vi "CélulaDessalinizadora3.0.vi"() -> ()   [LabVIEW 2014]
panel:
  in  "Adsorção":bool
  in  "OK Button":bool
  in  "Documento de Texto":path
  out "Tempo":dbl
  in  "Condutividade Máxima":dbl
  in  "NÚMERO DE CICLOS":dbl
  in  "Liga/Desliga":bool
  in  "Escolha: Porta Serial":refnum<visa-resource-name>="COM3"
  out "Dessorção":bool
  out "Adsorção":bool
  out "Single-Pass":bool
  out "Batch":bool
  in  "BATCH / SINGLE PASS":bool
  out "Potencial de Célula [mV]":dbl(graph)
  out "pH":dbl(graph)
  out "Condutividade [us/cm]":dbl(graph)
  in  "Selecionar caso":T1(tab)
  in  "TEMPO DE ADSOR敲O P":dbl
  in  "CONDUTIVIDADE \nMÍNIMA NA ADSORÇÃO P":dbl
  in  "TEMPO DE DESSOR敲O P":dbl
  in  "CONDUTIVIDADE \nMÁXIMA NA DESSORÇÃO P":dbl
  in  "Selecionar parâmetro G":enum32{"Tempo", "Condutividade", "Potencial"}(tab)
  in  "TEMPO DE ADSOR敲O G":dbl
  in  "TEMPO DE DESSOR敲O G":dbl
  in  "CONDUTIVIDADE \nMÍNIMA NA ADSORÇÃO G":dbl
  in  "CONDUTIVIDADE \nMÁXIMA NA DESSORÇÃO G":dbl
  in  "POTENCIAL DE CORTE\nNA ADSOR敲O":dbl
  in  "POTENCIAL DE CORTE\nNA DESSOR敲O":dbl
  in  "POTENCIAL DE CORTE\nNA DESSOR敲O G":dbl
  in  "CONDUTIVIDADE \nMÁXIMA NA DESSORÇÃO G2":dbl
  in  "TEMPO DE DESSOR敲O G 2":dbl
  in  "TEMPO DE ADSOR敲O G 2":dbl
  in  "CONDUTIVIDADE \nMÍNIMA NA ADSORÇÃO G 2":dbl
  in  "POTENCIAL DE CORTE\nNA ADSOR敲O G":dbl
  # "CONDUTIVIDADE MÁXIMA"
  # "s"
  # "us/cm"
  # "s"
  # "us/cm"
  # "s"
  # "s"
  # "us/cm"
  # "us/cm"
  # "VV"
  # "V"
  # "s"
  # "us/cm"
  # "mV"
  # "s"
  # "us/cm"
  # "mV"
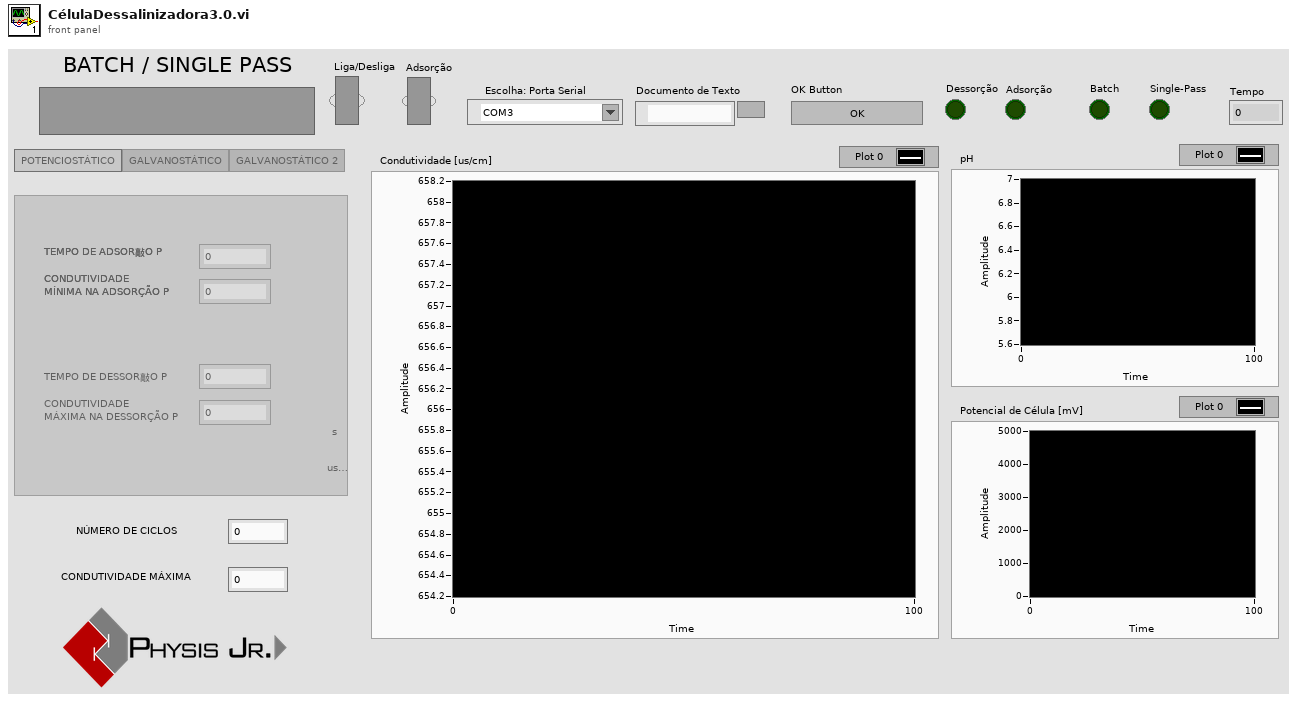
[diagram p1: front panel]
types:
  T1 = enum32{"POTENCIOSTÁTICO", "GALVANOSTÁTICO", "GALVANOSTÁTICO 2"}
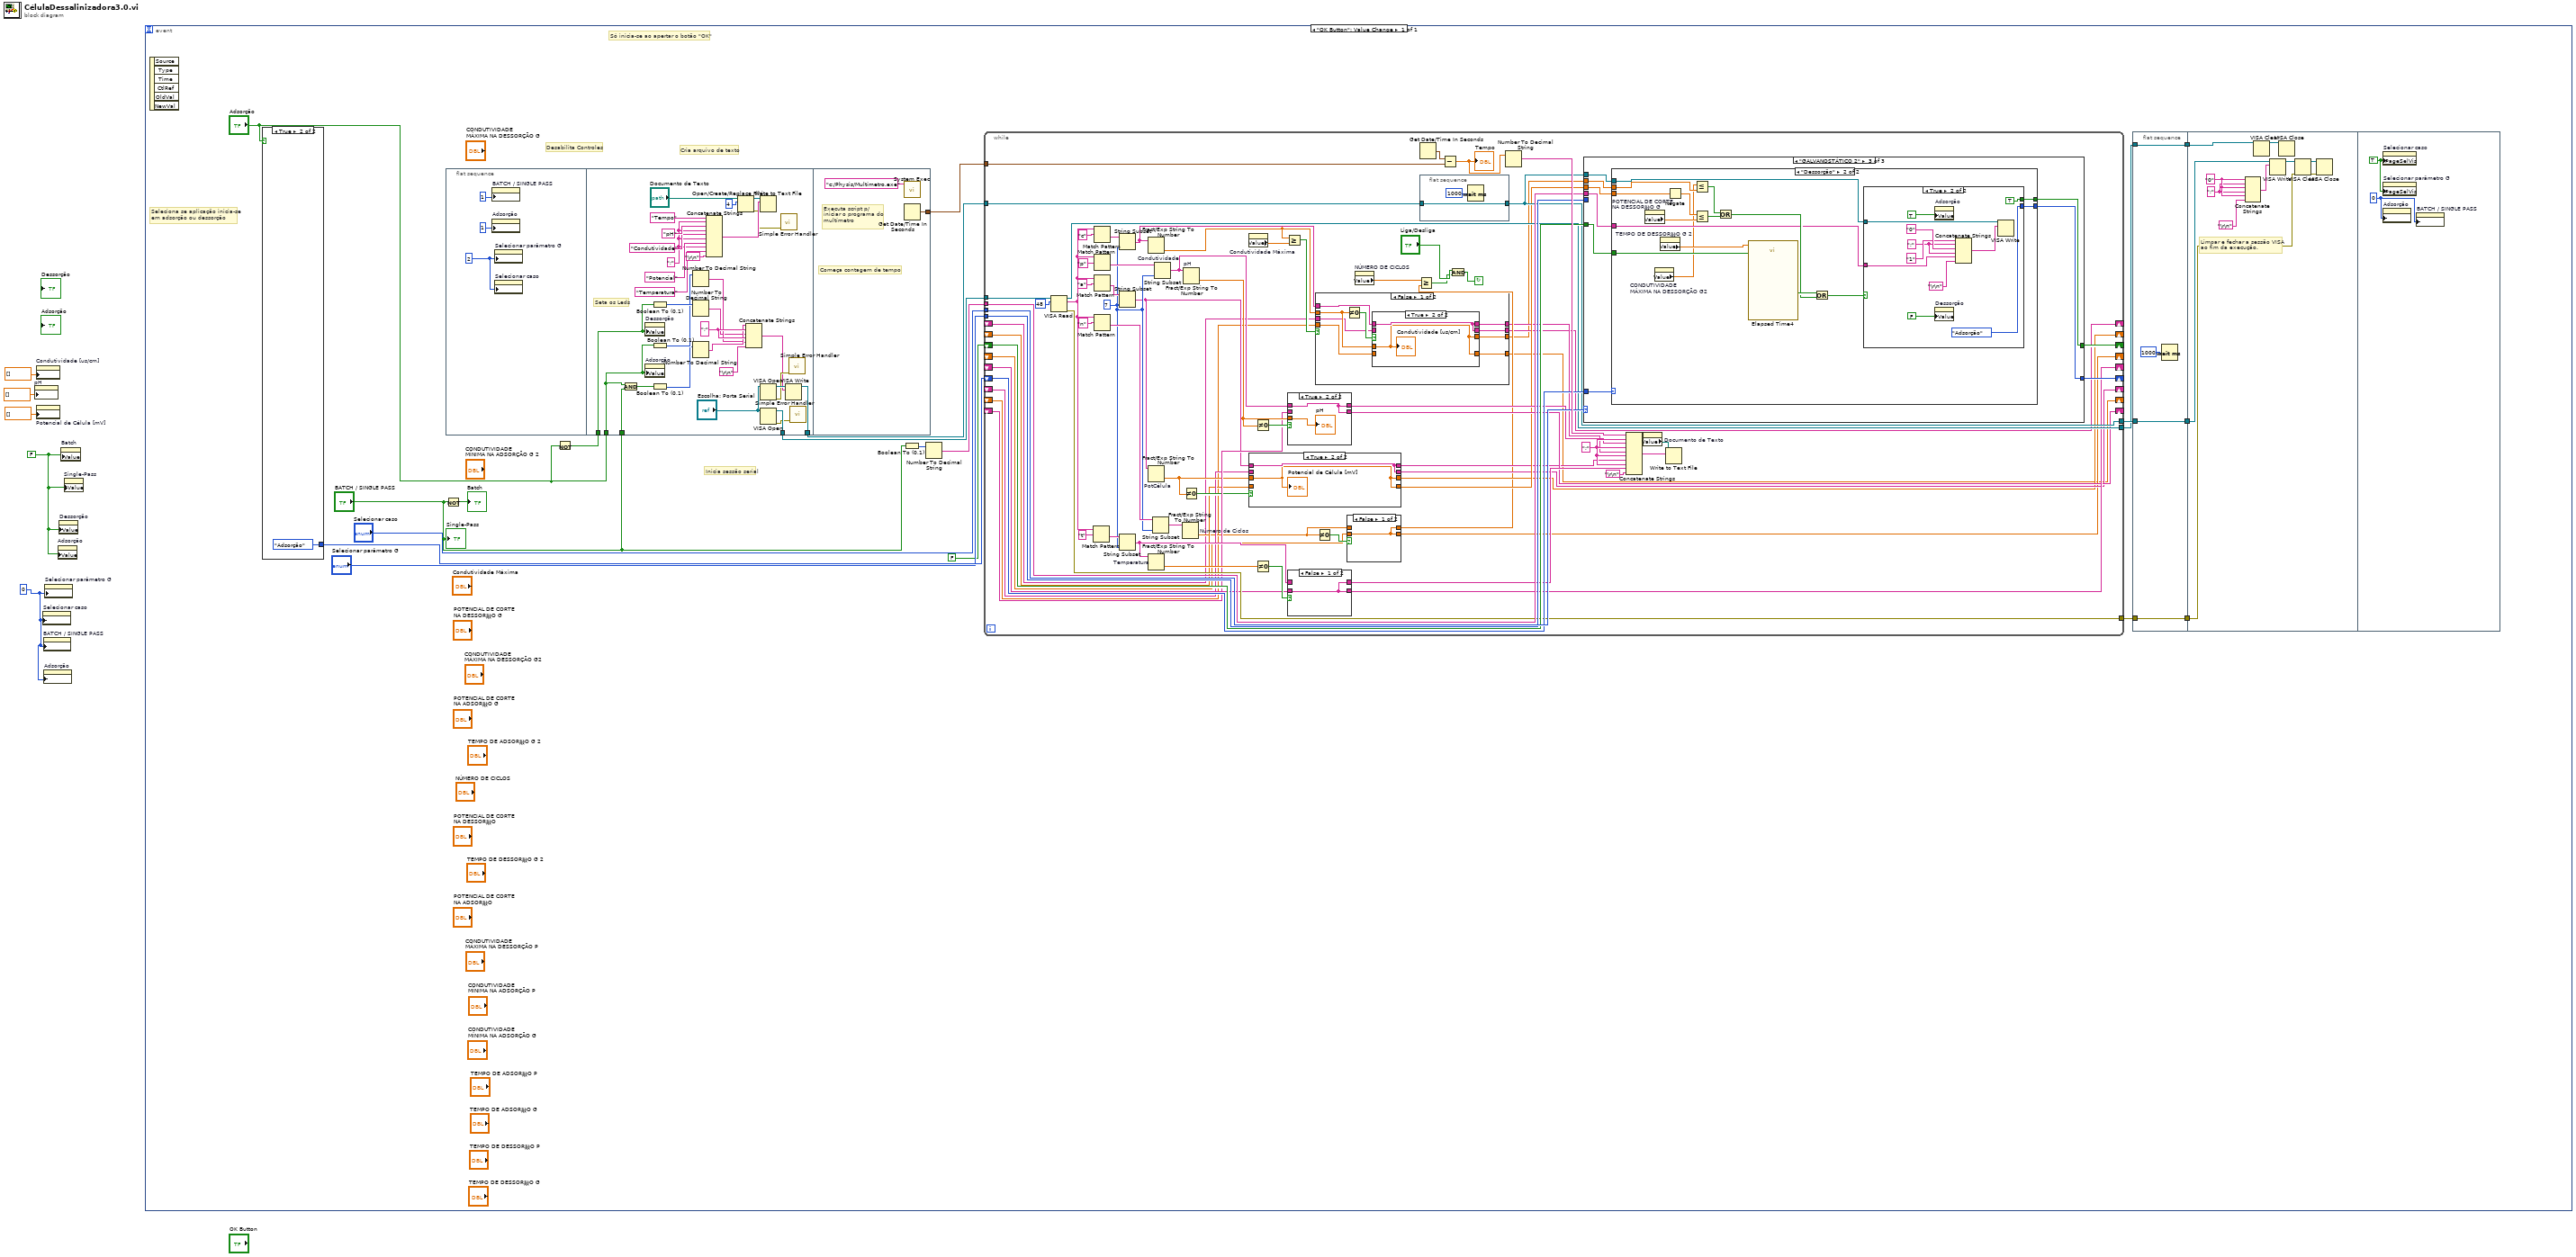
[diagram p0: block diagram]
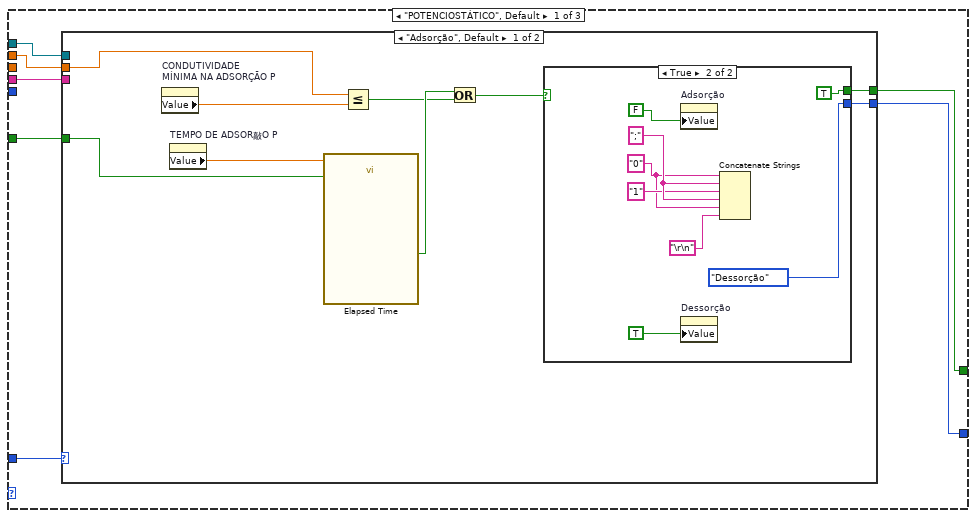
[diagram p6: hidden frame]
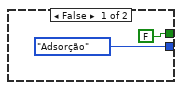
[diagram p7: hidden frame]
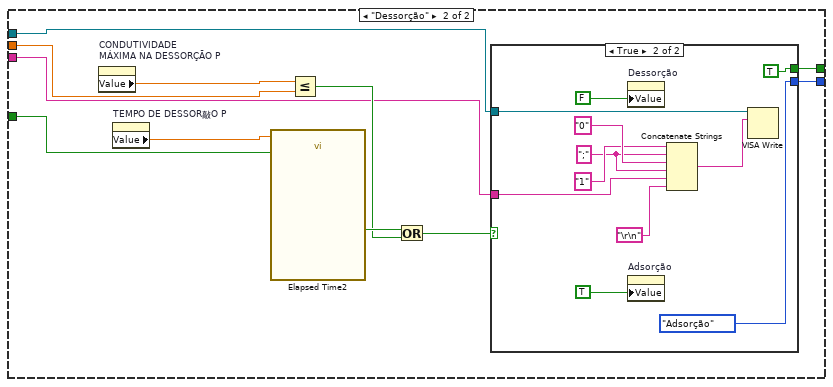
[diagram p8: hidden frame]
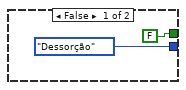
[diagram p9: hidden frame]
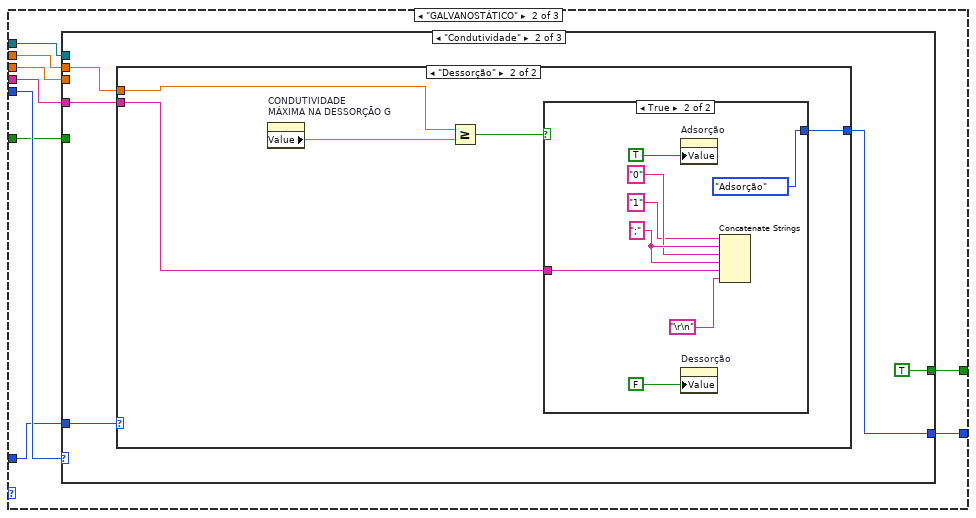
[diagram p10: hidden frame]
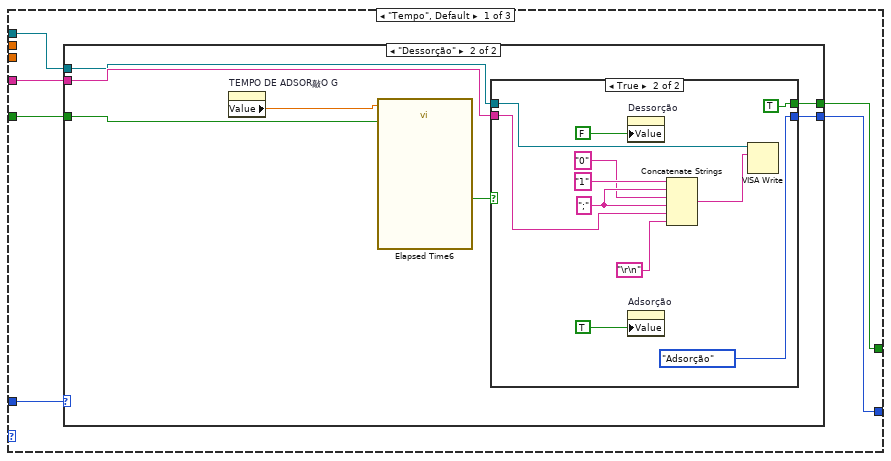
[diagram p11: hidden frame]
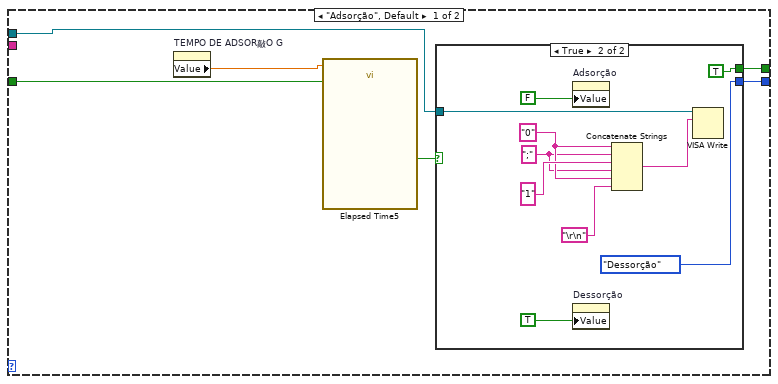
[diagram p12: hidden frame]
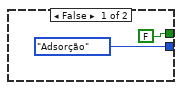
[diagram p13: hidden frame]
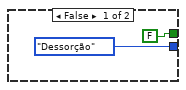
[diagram p14: hidden frame]
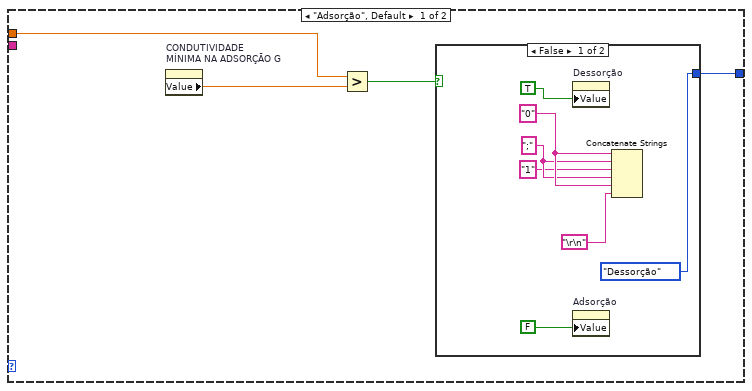
[diagram p15: hidden frame]
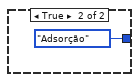
[diagram p16: hidden frame]
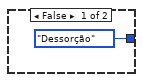
[diagram p17: hidden frame]
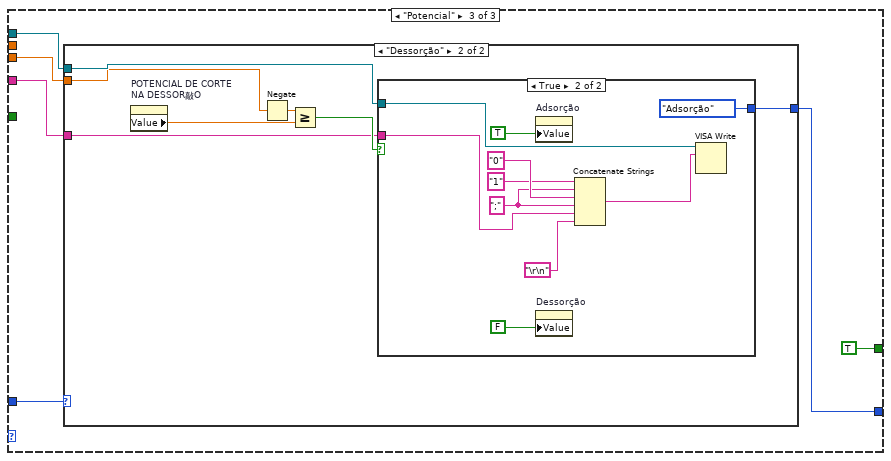
[diagram p18: hidden frame]
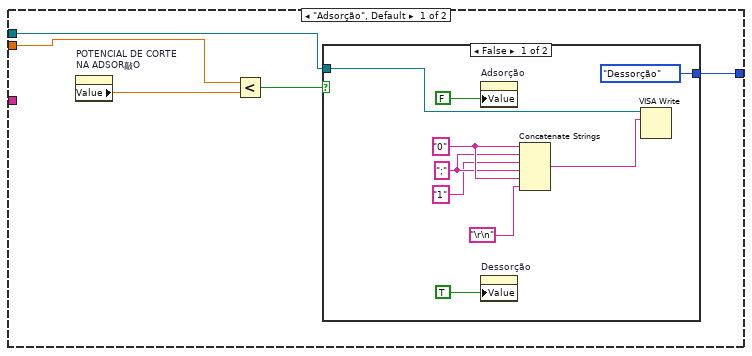
[diagram p19: hidden frame]
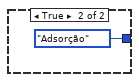
[diagram p20: hidden frame]
diagram:
  w1 = 0
  w2 = FALSE
  n1 = property on="pH" class="WFChart (strict)"("History Data"=dbl[] []) -> ()  [unwired: 2 in, 2 out]
  n2 = property on="Condutividade [us/cm]" class="WFChart (strict)"("History Data"=dbl[] []) -> ()  [unwired: 2 in, 2 out]
  n3 = property on="Potencial de Célula [mV]" class="WFChart (strict)"("History Data"=dbl[] []) -> ()  [unwired: 2 in, 2 out]
  n4 = property on="Selecionar caso" class="TabCtl (strict)"("DisabledEnum"=w1) -> ()  [unwired: 2 in, 2 out]
  n5 = property on="BATCH / SINGLE PASS" class="Bool (strict)"("DisabledEnum"=w1) -> ()  [unwired: 2 in, 2 out]
  n6 = property on="Adsorção" class="Bool (strict)"("DisabledEnum"=w1) -> ()  [unwired: 2 in, 2 out]
  n7 = property on="Selecionar parâmetro G" class="TabCtl (strict)"("DisabledEnum"=w1) -> ()  [unwired: 2 in, 2 out]
  n8 = property on="Adsorção" class="Bool (strict)"("Value"=w2) -> ()  [unwired: 2 in, 2 out]
  n9 = property on="Dessorção" class="Bool (strict)"("Value"=w2) -> ()  [unwired: 2 in, 2 out]
  n10 = property on="Batch" class="Bool (strict)"("Value"=w2) -> ()  [unwired: 2 in, 2 out]
  n11 = property on="Single-Pass" class="Bool (strict)"("Value"=w2) -> ()  [unwired: 2 in, 2 out]
  n12 = event shown="[0] \"OK Button\": Value Change" {
    selector: _ -> [_]
    dyn-events: _ -> [_]
    timeout: _ -> [_]
    event "OK Button": Value Change {
      # "Inicia sessão serial"
      # "Cria arquivo de texto"
      # "Desabilita Controles"
      # "Só inicia-se ao apertar o botão \"OK\""
      # "Seleciona se aplicação inicia-se\nem adsorção ou dessorção"
      n13 = event-data() -> ()  [unwired: 1 in, 6 out]
      n14 = case shown="True" "Adsorção" {
        tunnel: [enum16{"Adsorção", "Dessorção"}."Dessorção" enum16{"Adsorção", "Dessorção"}."Adsorção"] -> w18
        frame False {
        }
        frame True {
        }
      }
      n15 = Not(x="BATCH / SINGLE PASS") -> (.not. x?=→"Batch":bool)
      n16 = flat-sequence {
        tunnel: "Adsorção" -> [w47]
        tunnel: w16 -> [w56]
        tunnel: "BATCH / SINGLE PASS" -> [w59]
        tunnel: [w55] -> w11
        tunnel: [w54] -> w10
        tunnel: [w77] -> w15
        frame #0 {
          w42 = 2
          n17 = property on="BATCH / SINGLE PASS" class="Bool (strict)"("DisabledEnum"=1) -> ()  [unwired: 2 in, 2 out]
          n18 = property on="Adsorção" class="Bool (strict)"("DisabledEnum"=1) -> ()  [unwired: 2 in, 2 out]
          n19 = property on="Selecionar parâmetro G" class="TabCtl (strict)"("DisabledEnum"=w42) -> ()  [unwired: 2 in, 2 out]
          n20 = property on="Selecionar caso" class="TabCtl (strict)"("DisabledEnum"=w42) -> ()  [unwired: 2 in, 2 out]
        }
        frame #1 {
          w63 = ";"
          w67 = ";"
          # "Seta os Leds"
          n21 = And(x=w47, y=w59) -> (x .and. y?=w58:bool)
          n22 = property on="Dessorção" class="Bool (strict)"("Value"=w56) -> ()  [unwired: 2 in, 2 out]
          n23 = property on="Adsorção" class="Bool (strict)"("Value"=w47) -> ()  [unwired: 2 in, 2 out]
          n24 = Boolean To (0,1)(Boolean=w56) -> (0, 1=w61:i16)
          n25 = Boolean To (0,1)(Boolean=w47) -> (0, 1=w60:i16)
          n26 = Boolean To (0,1)(Boolean=w58) -> (0, 1=w57:i16)
          n27 = Number To Decimal String(number=w60) -> (decimal integer string=w49:string)  [unwired: 1 in]
          n28 = Number To Decimal String(number=w61) -> (decimal integer string=w48:string)  [unwired: 1 in]
          n29 = Number To Decimal String(number=w57) -> (decimal integer string=w50:string)  [unwired: 1 in]
          n30 = Concatenate Strings("Tempo", w67, "pH", w67, "Condutividade", w67, "Potencial", w67, "Temperatura", "\r\n") -> (w65:string)
          n31 = Open/Create/Replace File(file path (use dialog)="Documento de Texto", operation (0:open)=4) -> (refnum out=w73:refnum<file>, error out=w53:errorcluster)  [unwired: 4 in, 1 out]
          n32 = Concatenate Strings(w50, w63, w48, w63, w49, "\r\n") -> (w46:string)
          n33 = Write to Text File(file (use dialog)=w73, text=w65) -> ()  [unwired: 2 in, 3 out]
          n34 = VISA Open(VISA resource name="Escolha: Porta Serial") -> (VISA resource name=w62:refnum<visa-resource-name>, error out=w52:errorcluster)  [unwired: 4 in]
          n35 = VISA Open(VISA resource name="Escolha: Porta Serial") -> (VISA resource name=w55:refnum<visa-resource-name>, error out=w51:errorcluster)  [unwired: 4 in]
          n36 = call <vilib>:"Simple Error Handler.vi"("error in (no error)"=w53) -> ()  [unwired: 4 in, 5 out]
          n37 = VISA Write(VISA resource name=w62, write buffer=w46) -> (VISA resource name out=w54:refnum<visa-resource-name>)  [unwired: 1 in, 2 out]
          n38 = call <vilib>:"Simple Error Handler.vi"("error in (no error)"=w52) -> ()  [unwired: 4 in, 5 out]
          n39 = call <vilib>:"Simple Error Handler.vi"("error in (no error)"=w51) -> ()  [unwired: 4 in, 5 out]
        }
        frame #2 {
          # "Executa script p/\niniciar o programa do\nmultímetro"
          # "Começa contagem de tempo"
          n40 = call <vilib>:"System Exec.vi"("command line"="c:/Physis/Multímetro.exe") -> ()  [unwired: 7 in, 4 out]
          n41 = Get Date/Time In Seconds() -> (seconds since 1Jan1904=w77:timestamp)
        }
      }
      n42 = Not(x="Adsorção") -> (.not. x?=w16:bool)
      n43 = Boolean To (0,1)(Boolean="BATCH / SINGLE PASS") -> (0, 1=w13:i16)
      n44 = Number To Decimal String(number=w13) -> (decimal integer string=w12:string)  [unwired: 1 in]
      n45 = while {
        tunnel: w11 -> [w150]
        tunnel: w15 -> [w128]
        tunnel: "Selecionar caso" -> [w127]
        shift-right: [w126] -> _
        shift-left: w18 -> [w125]
        shift-right: [w124] -> _
        shift-left: FALSE -> [w123]
        tunnel: w12 -> [w122]
        tunnel: w10 -> [w120]
        tunnel: "Selecionar parâmetro G" -> [w121]
        tunnel: [w119] -> w9
        tunnel: [w118] -> w8
        tunnel: [w117] -> w7
        shift-right: [w110] -> _
        shift-left: _ -> [w109]
        shift-right: [w104] -> _
        shift-left: _ -> [w103]
        shift-right: [w97] -> _
        shift-left: _ -> [w96]
        shift-right: [w95] -> _
        shift-left: _ -> [w94]
        shift-right: [w90] -> _
        shift-left: _ -> [w89]
        shift-right: [w86] -> _
        shift-left: _ -> [w85]
        shift-right: [w83] -> _
        shift-left: _ -> [w82]
        stop <- w78 continue-if-true
        w132 = ";"
        w139 = 7
        n46 = VISA Read(VISA resource name=w150, byte count=48) -> (VISA resource name out=w118:refnum<visa-resource-name>, read buffer=w137:string, error out=w117:errorcluster)  [unwired: 1 in, 1 out]
        n47 = Match Pattern(string=w137, regular expression="t") -> (after substring=w145:string)  [unwired: 1 in, 3 out]
        n48 = Match Pattern(string=w137, regular expression="c") -> (after substring=w140:string)  [unwired: 1 in, 3 out]
        n49 = Match Pattern(string=w137, regular expression="a") -> (after substring=w143:string)  [unwired: 1 in, 3 out]
        n50 = Match Pattern(string=w137, regular expression="p") -> (after substring=w144:string)  [unwired: 1 in, 3 out]
        n51 = Match Pattern(string=w137, regular expression="n") -> (after substring=w142:string)  [unwired: 1 in, 3 out]
        n52 = String Subset(string=w140, length (rest)=w139) -> (substring=w129:string)  [unwired: 1 in]
        n53 = String Subset(string=w143, length (rest)=w139) -> (substring=w99:string)  [unwired: 1 in]
        n54 = String Subset(string=w145, length (rest)=w139) -> (substring=w112:string)  [unwired: 1 in]
        n55 = Fract/Exp String To Number "Condutividade"(string=w129) -> (number=w88:dbl)  [unwired: 3 in, 1 out]
        n56 = Fract/Exp String To Number "PotCélula"(string=w99) -> (number=w101:dbl)  [unwired: 3 in, 1 out]
        n57 = Fract/Exp String To Number "Temperatura"(string=w112) -> (number=w114:dbl)  [unwired: 3 in, 1 out]
        n58 = String Subset(string=w142, length (rest)=w139) -> (substring=w138:string)  [unwired: 1 in]
        n59 = String Subset(string=w144, length (rest)=w139) -> (substring=w106:string)  [unwired: 1 in]
        n60 = Fract/Exp String To Number "Número de Ciclos"(string=w138) -> (number=w92:dbl)  [unwired: 3 in, 1 out]
        n61 = Fract/Exp String To Number "pH"(string=w106) -> (number=w107:dbl)  [unwired: 3 in, 1 out]
        n62 = Not Equal To 0?(x=w101) -> (x != 0?=w102:bool)
        n63 = property on="Condutividade Máxima" class="DigNum (strict)"() -> ("Value"=w116:dbl)  [unwired: 2 in, 2 out]
        n64 = case shown="True" w102 {
          tunnel: w101 -> [_ w156]
          tunnel: [w154 w156] -> w100
          tunnel: w99 -> [_ w157]
          tunnel: [w155 w157] -> w98
          tunnel: [w155 w157] -> w97
          tunnel: w96 -> [w155 _]
          tunnel: [w154 w156] -> w95
          tunnel: w94 -> [w154 _]
          frame False {
          }
          frame True {
            "Potencial de Célula [mV]" <- w156
          }
        }
        n65 = Not Equal To 0?(x=w107) -> (x != 0?=w108:bool)
        n66 = Not Equal To 0?(x=w114) -> (x != 0?=w113:bool)
        n67 = Greater Or Equal?(x=w88, y=w116) -> (x >= y?=w130:bool)
        n68 = case shown="True" w108 {
          tunnel: w107 -> [_ w160]
          tunnel: w106 -> [_ w159]
          tunnel: [w158 w159] -> w105
          tunnel: [w158 w159] -> w104
          tunnel: w103 -> [w158 _]
          frame False {
          }
          frame True {
            "pH" <- w160
          }
        }
        n69 = case shown="False" w113 {
          tunnel: w112 -> [_ w162]
          tunnel: [w161 w162] -> w111
          tunnel: [w161 w162] -> w110
          tunnel: w109 -> [w161 _]
          frame False {
          }
          frame True {
          }
        }
        n70 = case shown="False" w130 {
          tunnel: w129 -> [w406 _]
          tunnel: w88 -> [w408 _]
          tunnel: [w407 w415] -> w87
          tunnel: [w405 w415] -> w86
          tunnel: w85 -> [w404 w415]
          tunnel: [w403 w414] -> w84
          tunnel: [w402 w414] -> w83
          tunnel: w82 -> [w401 w414]
          frame False {
            n71 = Not Equal To 0?(x=w408) -> (x != 0?=w409:bool)
            n72 = case shown="True" w409 {
              tunnel: w408 -> [_ w412]
              tunnel: [w411 w413] -> w407
              tunnel: w406 -> [_ w413]
              tunnel: [w411 w413] -> w405
              tunnel: w404 -> [w411 _]
              tunnel: [w410 w412] -> w403
              tunnel: [w410 w412] -> w402
              tunnel: w401 -> [w410 _]
              frame False {
              }
              frame True {
                "Condutividade [us/cm]" <- w412
              }
            }
          }
          frame True {
          }
        }
        n73 = Not Equal To 0?(x=w92) -> (x != 0?=w93:bool)
        n74 = case shown="False" w93 {
          tunnel: w92 -> [_ w153]
          tunnel: [w152 w153] -> w91
          tunnel: [w152 w153] -> w90
          tunnel: w89 -> [w152 _]
          frame False {
          }
          frame True {
          }
        }
        n75 = property on="NÚMERO DE CICLOS" class="DigNum (strict)"() -> ("Value"=w115:dbl)  [unwired: 2 in, 2 out]
        n76 = Greater Or Equal?(x=w115, y=w91) -> (x >= y?=w79:bool)
        n77 = Get Date/Time In Seconds() -> (seconds since 1Jan1904=w136:timestamp)
        n78 = flat-sequence {
          tunnel: [w163] -> w119
          tunnel: w120 -> [w163]
          frame #0 {
            n79 = Wait (ms)(milliseconds to wait=1000) -> ()  [unwired: 1 out]
          }
        }
        n80 = Subtract(x=w136, y=w128) -> (x-y=w135:dbl)
        "Tempo" <- w135
        n81 = And(x="Liga/Desliga", y=w79) -> (x .and. y?=w78:bool)
        n82 = Number To Decimal String(number=w135) -> (decimal integer string=w133:string)  [unwired: 1 in]
        n83 = case shown="\"GALVANOSTÁTICO 2\"" w127 {
          tunnel: w84 -> [w165 w216 w343]
          tunnel: [w171 w220 w341] -> w126
          tunnel: w125 -> [w168 w222 w345]
          tunnel: [w170 w219 w340] -> w124
          tunnel: w123 -> [w169 w221 w344]
          tunnel: w122 -> [w167 w217 w338]
          tunnel: w100 -> [_ w215 w342]
          tunnel: w119 -> [w166 w218 w339]
          tunnel: w121 -> [_ w223 _]
          frame "POTENCIOSTÁTICO", Default {
            n84 = case shown="\"Adsorção\", Default" w168 {
              tunnel: w165 -> [w180 w200]
              tunnel: [w176 w196] -> w171
              tunnel: [w175 w195] -> w170
              tunnel: w169 -> [w174 w201]
              tunnel: w167 -> [_ w194]
              tunnel: w166 -> [_ w193]
              frame "Adsorção", Default {
                n85 = property on="CONDUTIVIDADE \nMÍNIMA NA ADSORÇÃO P" class="DigNum (strict)"() -> ("Value"=w173:dbl)  [unwired: 2 in, 2 out]
                n86 = property on="TEMPO DE ADSOR敲O P" class="DigNum (strict)"() -> ("Value"=w172:dbl)  [unwired: 2 in, 2 out]
                n87 = call "Elapsed Time"("Time Target (s)"=w172, "Reset"=w174) -> ("Time has Elapsed"=w179:bool)  [unwired: 10 in, 7 out]
                n88 = Less Or Equal?(x=w180, y=w173) -> (x <= y?=w178:bool)
                n89 = Or(x=w179, y=w178) -> (x .or. y?=w177:bool)
                n90 = case shown="True" w177 {
                  tunnel: [enum16{"Adsorção", "Dessorção"}."Adsorção" enum16{"Adsorção", "Dessorção"}."Dessorção"] -> w176
                  tunnel: [FALSE TRUE] -> w175
                  frame False {
                  }
                  frame True {
                    w183 = "0"
                    w186 = ";"
                    n91 = property on="Adsorção" class="Bool (strict)"("Value"=FALSE) -> ()  [unwired: 2 in, 2 out]
                    n92 = property on="Dessorção" class="Bool (strict)"("Value"=TRUE) -> ()  [unwired: 2 in, 2 out]
                    n93 = Concatenate Strings(w183, w186, "1", w186, w183, "\r\n") -> ()  [unwired: 1 out]
                  }
                }
              }
              frame "Dessorção" {
                n94 = property on="CONDUTIVIDADE \nMÁXIMA NA DESSORÇÃO P" class="DigNum (strict)"() -> ("Value"=w191:dbl)  [unwired: 2 in, 2 out]
                n95 = property on="TEMPO DE DESSOR敲O P" class="DigNum (strict)"() -> ("Value"=w192:dbl)  [unwired: 2 in, 2 out]
                n96 = call "Elapsed Time2"("Time Target (s)"=w192, "Reset"=w201) -> ("Time has Elapsed"=w199:bool)  [unwired: 10 in, 7 out]
                n97 = Less Or Equal?(x=w191, y=w200) -> (x <= y?=w198:bool)
                n98 = Or(x=w199, y=w198) -> (x .or. y?=w197:bool)
                n99 = case shown="True" w197 {
                  tunnel: [enum16{"Adsorção", "Dessorção"}."Dessorção" enum16{"Adsorção", "Dessorção"}."Adsorção"] -> w196
                  tunnel: [FALSE TRUE] -> w195
                  tunnel: w194 -> [_ w209]
                  tunnel: w193 -> [_ w207]
                  frame False {
                  }
                  frame True {
                    w205 = ";"
                    n100 = property on="Dessorção" class="Bool (strict)"("Value"=FALSE) -> ()  [unwired: 2 in, 2 out]
                    n101 = property on="Adsorção" class="Bool (strict)"("Value"=TRUE) -> ()  [unwired: 2 in, 2 out]
                    n102 = Concatenate Strings("1", w205, "0", w205, w209, "\r\n") -> (w206:string)
                    n103 = VISA Write(VISA resource name=w207, write buffer=w206) -> ()  [unwired: 1 in, 3 out]
                  }
                }
              }
            }
          }
          frame "GALVANOSTÁTICO" {
            n104 = case shown="\"Condutividade\"" w223 {
              tunnel: w222 -> [w229 w272 w303]
              tunnel: w221 -> [w228 _ _]
              tunnel: [w227 w270 w301] -> w220
              tunnel: [w226 TRUE TRUE] -> w219
              tunnel: w218 -> [w225 _ w300]
              tunnel: w217 -> [w224 w268 w299]
              tunnel: w216 -> [_ w271 _]
              tunnel: w215 -> [_ _ w302]
              frame "Tempo", Default {
                n105 = case shown="\"Dessorção\"" w229 {
                  tunnel: w228 -> [w235 w254]
                  tunnel: [w233 w252] -> w227
                  tunnel: [w232 w251] -> w226
                  tunnel: w225 -> [w231 w249]
                  tunnel: w224 -> [_ w250]
                  frame "Adsorção", Default {
                    n106 = property on="TEMPO DE ADSOR敲O G" class="DigNum (strict)"() -> ("Value"=w230:dbl)  [unwired: 2 in, 2 out]
                    n107 = call "Elapsed Time5"("Time Target (s)"=w230, "Reset"=w235) -> ("Time has Elapsed"=w234:bool)  [unwired: 10 in, 7 out]
                    n108 = case shown="True" w234 {
                      tunnel: [enum16{"Adsorção", "Dessorção"}."Adsorção" enum16{"Adsorção", "Dessorção"}."Dessorção"] -> w233
                      tunnel: [FALSE TRUE] -> w232
                      tunnel: w231 -> [_ w240]
                      frame False {
                      }
                      frame True {
                        w242 = "0"
                        w239 = ";"
                        n109 = property on="Adsorção" class="Bool (strict)"("Value"=FALSE) -> ()  [unwired: 2 in, 2 out]
                        n110 = property on="Dessorção" class="Bool (strict)"("Value"=TRUE) -> ()  [unwired: 2 in, 2 out]
                        n111 = Concatenate Strings(w242, w239, "1", w239, w242, "\r\n") -> (w241:string)
                        n112 = VISA Write(VISA resource name=w240, write buffer=w241) -> ()  [unwired: 1 in, 3 out]
                      }
                    }
                  }
                  frame "Dessorção" {
                    n113 = property on="TEMPO DE ADSOR敲O G" class="DigNum (strict)"() -> ("Value"=w248:dbl)  [unwired: 2 in, 2 out]
                    n114 = call "Elapsed Time6"("Time Target (s)"=w248, "Reset"=w254) -> ("Time has Elapsed"=w253:bool)  [unwired: 10 in, 7 out]
                    n115 = case shown="True" w253 {
                      tunnel: [enum16{"Adsorção", "Dessorção"}."Dessorção" enum16{"Adsorção", "Dessorção"}."Adsorção"] -> w252
                      tunnel: [FALSE TRUE] -> w251
                      tunnel: w250 -> [_ w260]
                      tunnel: w249 -> [_ w258]
                      frame False {
                      }
                      frame True {
                        w263 = ";"
                        n116 = property on="Dessorção" class="Bool (strict)"("Value"=FALSE) -> ()  [unwired: 2 in, 2 out]
                        n117 = property on="Adsorção" class="Bool (strict)"("Value"=TRUE) -> ()  [unwired: 2 in, 2 out]
                        n118 = Concatenate Strings("1", w263, "0", w263, w260, "\r\n") -> (w259:string)
                        n119 = VISA Write(VISA resource name=w258, write buffer=w259) -> ()  [unwired: 1 in, 3 out]
                      }
                    }
                  }
                }
              }
              frame "Condutividade" {
                n120 = case shown="\"Dessorção\"" w272 {
                  tunnel: w271 -> [w276 w289]
                  tunnel: [w274 w287] -> w270
                  tunnel: w268 -> [_ w286]
                  frame "Adsorção", Default {
                    n121 = property on="CONDUTIVIDADE \nMÍNIMA NA ADSORÇÃO G" class="DigNum (strict)"() -> ("Value"=w273:dbl)  [unwired: 2 in, 2 out]
                    n122 = Greater?(x=w276, y=w273) -> (0:w275:bool)
                    n123 = case shown="False" w275 {
                      tunnel: [enum16{"Adsorção", "Dessorção"}."Dessorção" enum16{"Adsorção", "Dessorção"}."Adsorção"] -> w274
                      frame False {
                        w280 = "0"
                        w279 = ";"
                        n124 = property on="Dessorção" class="Bool (strict)"("Value"=TRUE) -> ()  [unwired: 2 in, 2 out]
                        n125 = property on="Adsorção" class="Bool (strict)"("Value"=FALSE) -> ()  [unwired: 2 in, 2 out]
                        n126 = Concatenate Strings(w280, w279, "1", w279, w280, "\r\n") -> ()  [unwired: 1 out]
                      }
                      frame True {
                      }
                    }
                  }
                  frame "Dessorção" {
                    n127 = property on="CONDUTIVIDADE \nMÁXIMA NA DESSORÇÃO G" class="DigNum (strict)"() -> ("Value"=w285:dbl)  [unwired: 2 in, 2 out]
                    n128 = Greater Or Equal?(x=w289, y=w285) -> (x >= y?=w288:bool)
                    n129 = case shown="True" w288 {
                      tunnel: [enum16{"Adsorção", "Dessorção"}."Dessorção" enum16{"Adsorção", "Dessorção"}."Adsorção"] -> w287
                      tunnel: w286 -> [_ w294]
                      frame False {
                      }
                      frame True {
                        w295 = ";"
                        n130 = property on="Adsorção" class="Bool (strict)"("Value"=TRUE) -> ()  [unwired: 2 in, 2 out]
                        n131 = property on="Dessorção" class="Bool (strict)"("Value"=FALSE) -> ()  [unwired: 2 in, 2 out]
                        n132 = Concatenate Strings("1", w295, "0", w295, w294, "\r\n") -> ()  [unwired: 1 out]
                      }
                    }
                  }
                }
              }
              frame "Potencial" {
                n133 = case shown="\"Dessorção\"" w303 {
                  tunnel: w302 -> [w305 w320]
                  tunnel: [w308 w325] -> w301
                  tunnel: w300 -> [w307 w323]
                  tunnel: w299 -> [_ w324]
                  frame "Adsorção", Default {
                    n134 = property on="POTENCIAL DE CORTE\nNA ADSOR敲O" class="DigNum (strict)"() -> ("Value"=w306:dbl)  [unwired: 2 in, 2 out]
                    n135 = Less?(x=w305, y=w306) -> (x < y?=w309:bool)
                    n136 = case shown="False" w309 {
                      tunnel: [enum16{"Adsorção", "Dessorção"}."Dessorção" enum16{"Adsorção", "Dessorção"}."Adsorção"] -> w308
                      tunnel: w307 -> [w316 _]
                      frame False {
                        w313 = "0"
                        w312 = ";"
                        n137 = property on="Adsorção" class="Bool (strict)"("Value"=FALSE) -> ()  [unwired: 2 in, 2 out]
                        n138 = property on="Dessorção" class="Bool (strict)"("Value"=TRUE) -> ()  [unwired: 2 in, 2 out]
                        n139 = Concatenate Strings(w313, w312, "1", w312, w313, "\r\n") -> (w317:string)
                        n140 = VISA Write(VISA resource name=w316, write buffer=w317) -> ()  [unwired: 1 in, 3 out]
                      }
                      frame True {
                      }
                    }
                  }
                  frame "Dessorção" {
                    n141 = property on="POTENCIAL DE CORTE\nNA DESSOR敲O" class="DigNum (strict)"() -> ("Value"=w322:dbl)  [unwired: 2 in, 2 out]
                    n142 = Negate(x=w320) -> (-x=w321:dbl)
                    n143 = Greater Or Equal?(x=w321, y=w322) -> (x >= y?=w326:bool)
                    n144 = case shown="True" w326 {
                      tunnel: [enum16{"Adsorção", "Dessorção"}."Dessorção" enum16{"Adsorção", "Dessorção"}."Adsorção"] -> w325
                      tunnel: w324 -> [_ w333]
                      tunnel: w323 -> [_ w331]
                      frame False {
                      }
                      frame True {
                        w330 = ";"
                        n145 = property on="Adsorção" class="Bool (strict)"("Value"=TRUE) -> ()  [unwired: 2 in, 2 out]
                        n146 = property on="Dessorção" class="Bool (strict)"("Value"=FALSE) -> ()  [unwired: 2 in, 2 out]
                        n147 = Concatenate Strings("1", w330, "0", w330, w333, "\r\n") -> (w332:string)
                        n148 = VISA Write(VISA resource name=w331, write buffer=w332) -> ()  [unwired: 1 in, 3 out]
                      }
                    }
                  }
                }
              }
            }
          }
          frame "GALVANOSTÁTICO 2" {
            n149 = case shown="\"Dessorção\"" w345 {
              tunnel: w344 -> [w359 w387]
              tunnel: w343 -> [w358 w386]
              tunnel: w342 -> [w357 w384]
              tunnel: [w351 w378] -> w341
              tunnel: [w350 w377] -> w340
              tunnel: w339 -> [w349 w376]
              tunnel: w338 -> [_ w375]
              frame "Adsorção", Default {
                n150 = property on="CONDUTIVIDADE \nMÍNIMA NA ADSORÇÃO G 2" class="DigNum (strict)"() -> ("Value"=w348:dbl)  [unwired: 2 in, 2 out]
                n151 = property on="POTENCIAL DE CORTE\nNA ADSOR敲O G" class="DigNum (strict)"() -> ("Value"=w347:dbl)  [unwired: 2 in, 2 out]
                n152 = property on="TEMPO DE ADSOR敲O G 2" class="DigNum (strict)"() -> ("Value"=w346:dbl)  [unwired: 2 in, 2 out]
                n153 = Less Or Equal?(x=w358, y=w348) -> (x <= y?=w356:bool)
                n154 = Less Or Equal?(x=w347, y=w357) -> (x <= y?=w355:bool)
                n155 = Or(x=w356, y=w355) -> (x .or. y?=w353:bool)
                n156 = call "Elapsed Time3"("Time Target (s)"=w346, "Reset"=w359) -> ("Time has Elapsed"=w354:bool)  [unwired: 10 in, 7 out]
                n157 = Or(x=w354, y=w353) -> (x .or. y?=w352:bool)
                n158 = case shown="True" w352 {
                  tunnel: [enum16{"Adsorção", "Dessorção"}."Adsorção" enum16{"Adsorção", "Dessorção"}."Dessorção"] -> w351
                  tunnel: [FALSE TRUE] -> w350
                  tunnel: w349 -> [_ w364]
                  frame False {
                  }
                  frame True {
                    w366 = "0"
                    w363 = ";"
                    n159 = property on="Adsorção" class="Bool (strict)"("Value"=FALSE) -> ()  [unwired: 2 in, 2 out]
                    n160 = property on="Dessorção" class="Bool (strict)"("Value"=TRUE) -> ()  [unwired: 2 in, 2 out]
                    n161 = Concatenate Strings(w366, w363, "1", w363, w366, "\r\n") -> (w365:string)
                    n162 = VISA Write(VISA resource name=w364, write buffer=w365) -> ()  [unwired: 1 in, 3 out]
                  }
                }
              }
              frame "Dessorção" {
                n163 = property on="POTENCIAL DE CORTE\nNA DESSOR敲O G" class="DigNum (strict)"() -> ("Value"=w373:dbl)  [unwired: 2 in, 2 out]
                n164 = property on="CONDUTIVIDADE \nMÁXIMA NA DESSORÇÃO G2" class="DigNum (strict)"() -> ("Value"=w372:dbl)  [unwired: 2 in, 2 out]
                n165 = property on="TEMPO DE DESSOR敲O G 2" class="DigNum (strict)"() -> ("Value"=w374:dbl)  [unwired: 2 in, 2 out]
                n166 = Negate(x=w384) -> (-x=w385:dbl)
                n167 = Less Or Equal?(x=w372, y=w386) -> (x <= y?=w383:bool)
                n168 = Less Or Equal?(x=w385, y=w373) -> (x <= y?=w382:bool)
                n169 = Or(x=w383, y=w382) -> (x .or. y?=w380:bool)
                n170 = call "Elapsed Time4"("Time Target (s)"=w374, "Reset"=w387) -> ("Time has Elapsed"=w381:bool)  [unwired: 10 in, 7 out]
                n171 = Or(x=w381, y=w380) -> (x .or. y?=w379:bool)
                n172 = case shown="True" w379 {
                  tunnel: [enum16{"Adsorção", "Dessorção"}."Dessorção" enum16{"Adsorção", "Dessorção"}."Adsorção"] -> w378
                  tunnel: [FALSE TRUE] -> w377
                  tunnel: w376 -> [_ w395]
                  tunnel: w375 -> [_ w392]
                  frame False {
                  }
                  frame True {
                    w391 = ";"
                    n173 = property on="Adsorção" class="Bool (strict)"("Value"=TRUE) -> ()  [unwired: 2 in, 2 out]
                    n174 = property on="Dessorção" class="Bool (strict)"("Value"=FALSE) -> ()  [unwired: 2 in, 2 out]
                    n175 = Concatenate Strings("1", w391, "0", w391, w392, "\r\n") -> (w396:string)
                    n176 = VISA Write(VISA resource name=w395, write buffer=w396) -> ()  [unwired: 1 in, 3 out]
                  }
                }
              }
            }
          }
        }
        n177 = Concatenate Strings(w133, w132, w105, w132, w87, w132, w98, w132, w111, "\r\n") -> (w134:string)
        n178 = property on="Documento de Texto" class="Path"() -> ("Value"=w81:path)  [unwired: 2 in, 2 out]
        n179 = Write to Text File(file (use dialog)=w81, text=w134) -> ()  [unwired: 2 in, 3 out]
      }
      n180 = flat-sequence {
        tunnel: w9 -> [w26]
        tunnel: w7 -> [w27]
        tunnel: w8 -> [w28]
        tunnel: [w28] -> w24
        tunnel: [w27] -> w23
        tunnel: [w26] -> w22
        tunnel: w24 -> [w34]
        tunnel: w23 -> [w33]
        tunnel: w22 -> [w31]
        frame #0 {
          n181 = Wait (ms)(milliseconds to wait=1000) -> ()  [unwired: 1 out]
        }
        frame #1 {
          w32 = "0"
          w30 = ";"
          # "Limpar e fechar a sessão VISA\nao fim da execução."
          n182 = Concatenate Strings(w32, w30, w32, w30, w32, "\r\n") -> (w38:string)
          n183 = VISA Clear(VISA resource name=w34) -> (VISA resource name out=w35:refnum<visa-resource-name>)  [unwired: 1 in, 1 out]
          n184 = VISA Write(VISA resource name=w31, write buffer=w38) -> (VISA resource name out=w39:refnum<visa-resource-name>)  [unwired: 1 in, 2 out]
          n185 = VISA Close(VISA resource name=w35) -> ()  [unwired: 1 in, 1 out]
          n186 = VISA Clear(VISA resource name=w39, error in (no error)=w33) -> (VISA resource name out=w36:refnum<visa-resource-name>, error out=w37:errorcluster)
          n187 = VISA Close(VISA resource name=w36, error in (no error)=w37) -> ()  [unwired: 1 out]
        }
        frame #2 {
          w40 = 0
          w41 = TRUE
          n188 = property on="Selecionar caso" class="TabCtl (strict)"("PageSelVis"=w41) -> ()  [unwired: 2 in, 2 out]
          n189 = property on="Selecionar parâmetro G" class="TabCtl (strict)"("PageSelVis"=w41) -> ()  [unwired: 2 in, 2 out]
          n190 = property on="Adsorção" class="Bool (strict)"("DisabledEnum"=w40) -> ()  [unwired: 2 in, 2 out]
          n191 = property on="BATCH / SINGLE PASS" class="Bool (strict)"("DisabledEnum"=w40) -> ()  [unwired: 2 in, 2 out]
        }
      }
      "Single-Pass" <- "BATCH / SINGLE PASS"
    }
  }
